vi "Teleop.vi"(10 "Match Info":T1={"Autonomous Elapsed Seconds"=0.0, "TeleOp Elapsed Seconds"=0.0, "Disabled Elapsed Seconds"=0.0, "Visited Autonomous"=FALSE, "Visited TeleOp"=FALSE, "Visited Disabled"=FALSE, "Autonomous Settings"={"Autonomous Style"=enum."Independent", "VI Refnum"=refnum}}, 11 "Call Context":T2) -> ()   [LabVIEW 2018]
doc: "This VI is called for each TeleOp packet received from the DS where the robot is not disabled. It is often used to read from the joysticks and update I/O or to update setpoints for timed control loops. It should complete and return within 20 milliseconds or it may miss DS packets."
uses:
  <vilib>/Rock Robotics/WPI/DriverStation/WPI_DriverStationDerivedRobotMode.ctl
  <vilib>/Rock Robotics/WPI/DriverStation/WPI_DriverStationMatch Info.ctl
  <vilib>/Rock Robotics/WPI/Utilities/WPI_GetSetVariantRefNum.vi
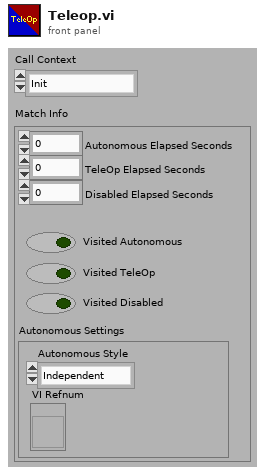
[diagram p1: front panel]
types:
  T1 = typedef "WPI_DriverStationMatch Info.ctl" = cluster{"Autonomous Elapsed Seconds":dbl, "TeleOp Elapsed Seconds":dbl, "Disabled Elapsed Seconds":dbl, "Visited Autonomous":bool, "Visited TeleOp":bool, "Visited Disabled":bool, "Autonomous Settings":cluster{"Autonomous Style":enum16{"Iterative", "Independent"}, "VI Refnum":refnum<vi>}}
  T2 = typedef "WPI_DriverStationDerivedRobotMode.ctl" = enum16{"Init", "Execute", "Stop"}
  T3 = typedef "WPI_JoystickDevRef.ctl" = cluster{"Device":T4}
  T4 = typedef "WPI_JoystickDeviceEnum.ctl" = enum16{"USB 0", "USB 1", "USB 2", "USB 3", "USB 4", "USB 5"}
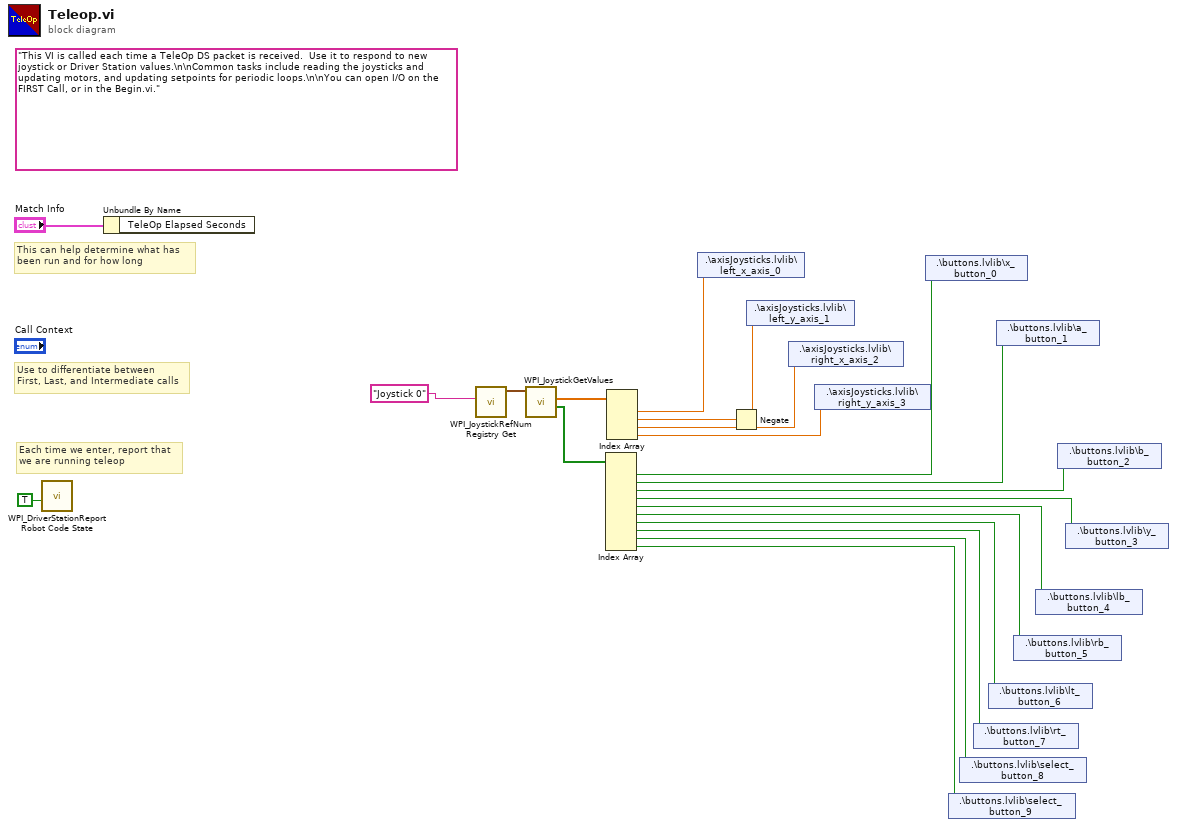
[diagram p0: block diagram]
diagram:
  (unwired) "This VI is called each time a TeleOp DS packet is received.  Use it to respond to new joystick or Driver Station values.\n\nCommon tasks include reading the joysticks and updating motors, and updating setpoints for periodic loops.\n\nYou can open I/O on the FIRST Call, or in the Begin.vi."
  # "Each time we enter, report that\nwe are running teleop"
  # "Use to differentiate between\nFirst, Last, and Intermediate calls"
  # "This can help determine what has\nbeen run and for how long"
  n1 = call <vilib>:"WPI_DriverStationReport Robot Code State.vi"("TeleOp"=TRUE ("Autonomous")) -> ()  [unwired: 10 in, 1 out]
  n2 = Unbundle By Name("Match Info") -> ()  [unwired: 1 out]
  n3 = call <vilib>:"WPI_JoystickRefNum Registry Get.vi"("refnum name"="Joystick 0") -> ("JoystickDevRef"=w20:T3)  [unwired: 1 in, 9 out]
  n4 = call <vilib>:"WPI_JoystickGetValues.vi"("JoystickDevRef"=w20) -> ("Buttons"=w17:bool[], "Axes"=w18:dbl[])  [unwired: 6 in, 3 out]
  n5 = Index Array(array=w17) -> (element #1=w16:bool, element #2=w15:bool, element #3=w14:bool, element #4=w13:bool, element #5=w12:bool, element #6=w11:bool, element #7=w10:bool, element #8=w9:bool, element #9=w8:bool, element #10=w7:bool)  [unwired: 10 in]
  n6 = Index Array(array=w18) -> (element #1=w6:dbl, element #2=w5:dbl, element #3=w4:dbl, element #4=w3:dbl)  [unwired: 4 in]
  n7 = shared-variable ".\\axisJoysticks.lvlib\\left_x_axis_0"(w6) -> ()  [unwired: 1 in, 1 out]
  n8 = Negate(x=w5) -> (-x=w1:dbl)
  n9 = shared-variable ".\\axisJoysticks.lvlib\\left_y_axis_1"(w1) -> ()  [unwired: 1 in, 1 out]
  n10 = shared-variable ".\\axisJoysticks.lvlib\\right_x_axis_2"(w4) -> ()  [unwired: 1 in, 1 out]
  n11 = shared-variable ".\\axisJoysticks.lvlib\\right_y_axis_3"(w3) -> ()  [unwired: 1 in, 1 out]
  n12 = shared-variable ".\\buttons.lvlib\\x_button_0"(w16) -> ()  [unwired: 1 in, 1 out]
  n13 = shared-variable ".\\buttons.lvlib\\select_button_9"(w7) -> ()  [unwired: 1 in, 1 out]
  n14 = shared-variable ".\\buttons.lvlib\\select_button_8"(w8) -> ()  [unwired: 1 in, 1 out]
  n15 = shared-variable ".\\buttons.lvlib\\rt_button_7"(w9) -> ()  [unwired: 1 in, 1 out]
  n16 = shared-variable ".\\buttons.lvlib\\lt_button_6"(w10) -> ()  [unwired: 1 in, 1 out]
  n17 = shared-variable ".\\buttons.lvlib\\a_button_1"(w15) -> ()  [unwired: 1 in, 1 out]
  n18 = shared-variable ".\\buttons.lvlib\\rb_button_5"(w11) -> ()  [unwired: 1 in, 1 out]
  n19 = shared-variable ".\\buttons.lvlib\\lb_button_4"(w12) -> ()  [unwired: 1 in, 1 out]
  n20 = shared-variable ".\\buttons.lvlib\\b_button_2"(w14) -> ()  [unwired: 1 in, 1 out]
  n21 = shared-variable ".\\buttons.lvlib\\y_button_3"(w13) -> ()  [unwired: 1 in, 1 out]
